vi "RenderTexture.vi"(4 "Dstrect":T1, 5 "Entire Rendering Target (F)":bool, 6 "Srcrect":T1, 7 "Entire Texture (F)":bool, 8 "No Error":errorcluster, 10 "Texture [SDL_Texture *]":i64 format="%.0x", 11 "Renderer [SDL_Renderer *]":i64 format="%.0x") -> (0 "error out":errorcluster)   [LabVIEW 2026, in "SDL3.lvlib" / "Render.lvlib"]
doc: "<B>Summary</B>\nCopy a portion of the texture to the current rendering target at subpixel precision."
uses:
  Render.lvlib
  Rect/FRect--cluster.ctl
  <vilib>/Utility/error.llb/Error Cluster From Error Code.vi
  Error/Error.lvlib
  Lib/SDL3.dll
  Rect/Rect.lvlib
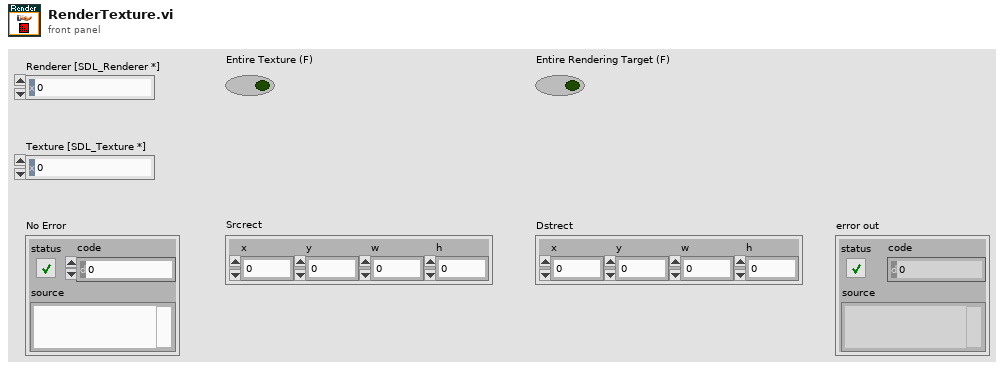
[diagram p1: front panel]
types:
  T1 = typedef "SDL3.lvlib/Rect.lvlib/FRect--cluster.ctl" = cluster{"x":sgl, "y":sgl, "w":sgl, "h":sgl}
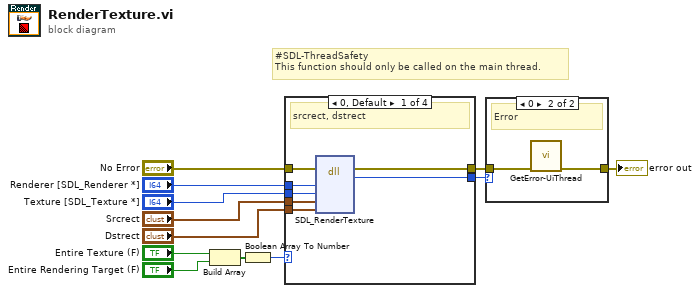
[diagram p0: block diagram]
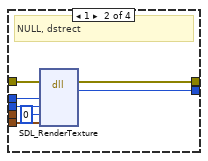
[diagram p2: hidden frame]
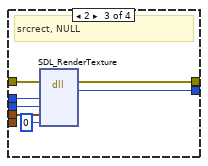
[diagram p3: hidden frame]
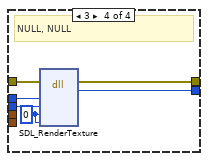
[diagram p4: hidden frame]
diagram:
  # "#SDL-ThreadSafety\nThis function should only be called on the main thread."
  n1 = Build Array("Entire Texture (F)", "Entire Rendering Target (F)") -> (w2:bool[])
  n2 = Boolean Array To Number(Boolean array=w2) -> (number=w1:u32)
  n3 = case shown="0, Default" w1 {
    tunnel: "No Error" -> [w19 w26 w33 w39]
    tunnel: [w18 w25 w32 w38] -> w4
    tunnel: [w17 w24 w31 w37] -> w3
    tunnel: "Renderer [SDL_Renderer *]" -> [w16 w23 w30 w36]
    tunnel: "Texture [SDL_Texture *]" -> [w15 w22 w29 w35]
    tunnel: "Srcrect" -> [w14 _ w28 _]
    tunnel: "Dstrect" -> [w13 w20 _ _]
    frame 0, Default {
      # "srcrect, dstrect"
      n4 = dll-call lib="C:/Users/saukko/Dev/LV-SDL3/Sources/SDL3/Lib/SDL3.*" fn="SDL_RenderTexture"(error in=w19, "renderer"=w16, "texture"=w15, "srcrect"=w14, "dstrect"=w13) -> (error out=w18:errorcluster, "return type"=w17:i32)  [unwired: 6 in, 1 out]
    }
    frame 1 {
      # "NULL, dstrect"
      n5 = dll-call lib="C:/Users/saukko/Dev/LV-SDL3/Sources/SDL3/Lib/SDL3.*" fn="SDL_RenderTexture"(error in=w26, "renderer"=w23, "texture"=w22, "srcrect"=i64 0 ("dstrect"), "dstrect"=w20) -> (error out=w25:errorcluster, "return type"=w24:i32)  [unwired: 6 in, 1 out]
    }
    frame 2 {
      # "srcrect, NULL"
      n6 = dll-call lib="C:/Users/saukko/Dev/LV-SDL3/Sources/SDL3/Lib/SDL3.*" fn="SDL_RenderTexture"(error in=w33, "renderer"=w30, "texture"=w29, "srcrect"=w28, "dstrect"=i64 0) -> (error out=w32:errorcluster, "return type"=w31:i32)  [unwired: 6 in, 1 out]
    }
    frame 3 {
      w34 = i64 0 ("dstrect")
      # "NULL, NULL"
      n7 = dll-call lib="C:/Users/saukko/Dev/LV-SDL3/Sources/SDL3/Lib/SDL3.*" fn="SDL_RenderTexture"(error in=w39, "renderer"=w36, "texture"=w35, "srcrect"=w34, "dstrect"=w34) -> (error out=w38:errorcluster, "return type"=w37:i32)  [unwired: 6 in, 1 out]
    }
  }
  n8 = case shown="0" w3 {
    tunnel: w4 -> [w40 w42]
    tunnel: [w40 w41] -> w11
    frame Default {
      # "Ok"
    }
    frame 0 {
      # "Error"
      n9 = call "GetError-UiThread.vi"("No Error"=w42) -> ("error out"=w41:errorcluster)  [unwired: 10 in]
    }
  }
  "error out" <- w11
